vi "DataArray_Reformatter.vi"(5 "Data Array":string[][](array[string])) -> (0 "MeltTemps":dbl[](array[numeric]), 1 "Offsets":dbl[](array[numeric]), 2 "FreezeTemps":dbl[](array[numeric]), 3 "Temps":dbl[][](graph), 4 "Offset Applied":bool)   [LabVIEW 2024]
panel:
  out "element":string
  out "FrozenFraction":dbl[](array[numeric])
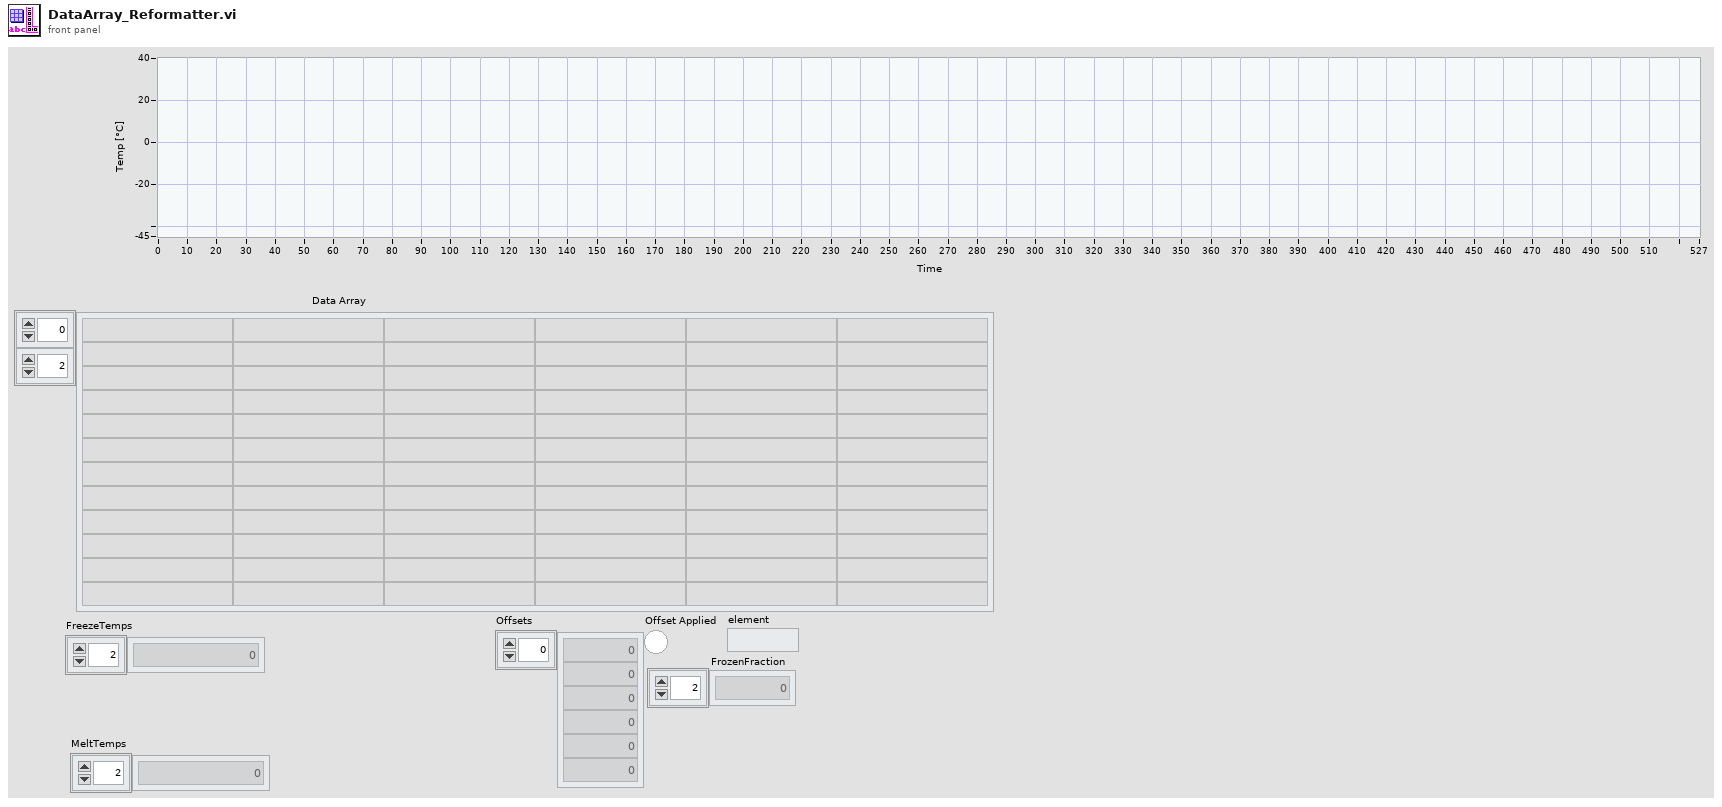
[diagram p1: front panel]
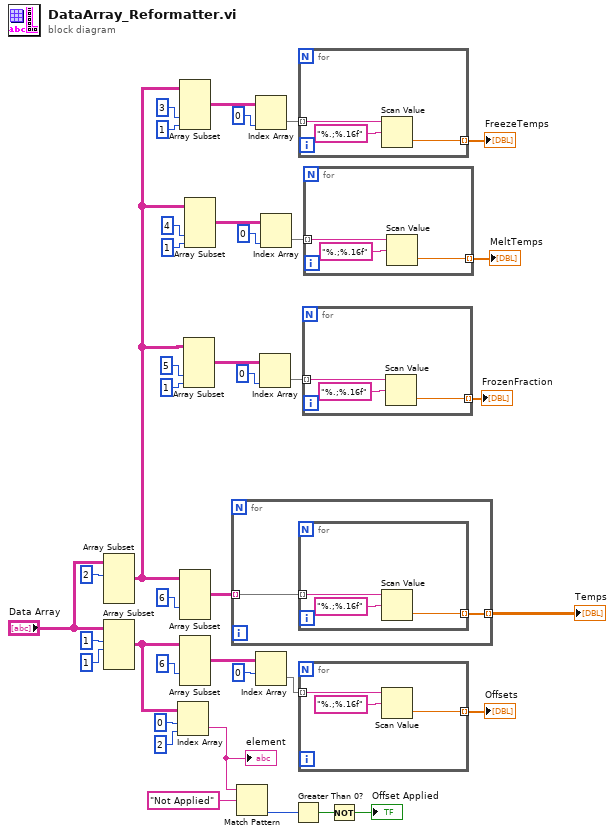
[diagram p0: block diagram]
diagram:
  n1 = Array Subset(array="Data Array", index (row)=2 ("index")) -> (w2:string[][])  [unwired: 3 in]
  n2 = Array Subset(array="Data Array", index (row)=1 ("index"), length (row)=1 ("length")) -> (w27:string[][])  [unwired: 2 in]
  n3 = Index Array(array=w27, index (row)=0 ("disabled index (col)"), index (col)=2 ("index (row)")) -> (element=w22:string)
  "element" <- w22
  n4 = Array Subset(array=w2, index (col)=3 ("index"), length (col)=1 ("length")) -> (w37:string[][])  [unwired: 2 in]
  n5 = Array Subset(array=w2, index (col)=6 ("index")) -> (w33:string[][])  [unwired: 3 in]
  n6 = Array Subset(array=w27, index (col)=6 ("index")) -> (w25:string[][])  [unwired: 3 in]
  n7 = Array Subset(array=w2, index (col)=5 ("index"), length (col)=1 ("length")) -> (w6:string[][])  [unwired: 2 in]
  n8 = Array Subset(array=w2, index (col)=4 ("index"), length (col)=1 ("length")) -> (w10:string[][])  [unwired: 2 in]
  n9 = for {
    tunnel: w33 -> [w41] mode=indexing
    tunnel: [w40] -> w8 mode=indexing
    n10 = for {
      tunnel: w41 -> [w43] mode=indexing
      tunnel: [w42] -> w40 mode=indexing
      n11 = Scan Value(string=w43, format string="%.;%.16f") -> (value=w42:dbl)  [unwired: 1 in, 1 out]
    }
  }
  "Temps" <- w8
  n12 = Match Pattern(string=w22, regular expression="Not Applied") -> (offset past match=w20:i32)  [unwired: 1 in, 3 out]
  n13 = Index Array(array=w37, index (col)=0 ("disabled index (col)")) -> (element=w32:string[])  [unwired: 1 in]
  n14 = Index Array(array=w25, index (row)=0 ("disabled index (col)")) -> (element=w24:string[])  [unwired: 1 in]
  n15 = Index Array(array=w6, index (col)=0 ("disabled index (col)")) -> (element=w3:string[])  [unwired: 1 in]
  n16 = Index Array(array=w10, index (col)=0 ("disabled index (col)")) -> (element=w13:string[])  [unwired: 1 in]
  n17 = Greater Than 0?(x=w20) -> (x > 0?=w19:bool)
  n18 = for {
    tunnel: w32 -> [w46] mode=indexing
    tunnel: [w45] -> w31 mode=indexing
    n19 = Scan Value(string=w46, format string="%.;%.16f") -> (value=w45:dbl)  [unwired: 1 in, 1 out]
  }
  "FreezeTemps" <- w31
  n20 = for {
    tunnel: w24 -> [w49] mode=indexing
    tunnel: [w48] -> w23 mode=indexing
    n21 = Scan Value(string=w49, format string="%.;%.16f") -> (value=w48:dbl)  [unwired: 1 in, 1 out]
  }
  "Offsets" <- w23
  n22 = for {
    tunnel: w3 -> [w52] mode=indexing
    tunnel: [w51] -> w1 mode=indexing
    n23 = Scan Value(string=w52, format string="%.;%.16f") -> (value=w51:dbl)  [unwired: 1 in, 1 out]
  }
  "FrozenFraction" <- w1
  n24 = for {
    tunnel: w13 -> [w55] mode=indexing
    tunnel: [w54] -> w14 mode=indexing
    n25 = Scan Value(string=w55, format string="%.;%.16f") -> (value=w54:dbl)  [unwired: 1 in, 1 out]
  }
  "MeltTemps" <- w14
  n26 = Not(x=w19) -> (.not. x?=→"Offset Applied":bool)
